vi "Create Plugin Groups.vi"(8 "error in (no error)":errorcluster, 10 "parent tag":string, 11 "Application Data In":T1) -> (0 "error out":errorcluster, 1 "async plugins tag":string, 2 "inline plugins tag":string, 3 "Application Data out":T1)   [LabVIEW 2017, in "DSF Core.lvlib"]
uses:
  DSF Core.lvlib
  Main VI/Application Data.ctl
  <vilib>/NI/Memory Manager/Classes/Pointer/Pointer.lvclass
  Classes/Framework/Framework.lvclass
  Buffer Reader/Buffer Data.ctl
  Classes/Buffer/Buffer.lvclass
  Classes/Transfer Group Status/Status.lvclass
  Typedefs/DSF Engine Framework Configuration.ctl
  Typedefs/DSF Engine Plugin Configuration.ctl
  Typedefs/DSF Timing Info.ctl
  Typedefs/DSF Engine Plugin Thread Configuration.ctl
  Typedefs/DSF Settings Info.ctl
  Typedefs/DSF Engine Transfer Group Configuration.ctl
  Typedefs/DSF Direction.ctl
  Typedefs/DSF Engine Transfer Configuration.ctl
  Typedefs/DSF Byte Order.ctl
  Typedefs/DSF Engine Channel Configuration.ctl
  Typedefs/DSF Data Type.ctl
  Typedefs/DSF Timeout Behavior.ctl
  ID to Tree Items/Tree Item Type.ctl
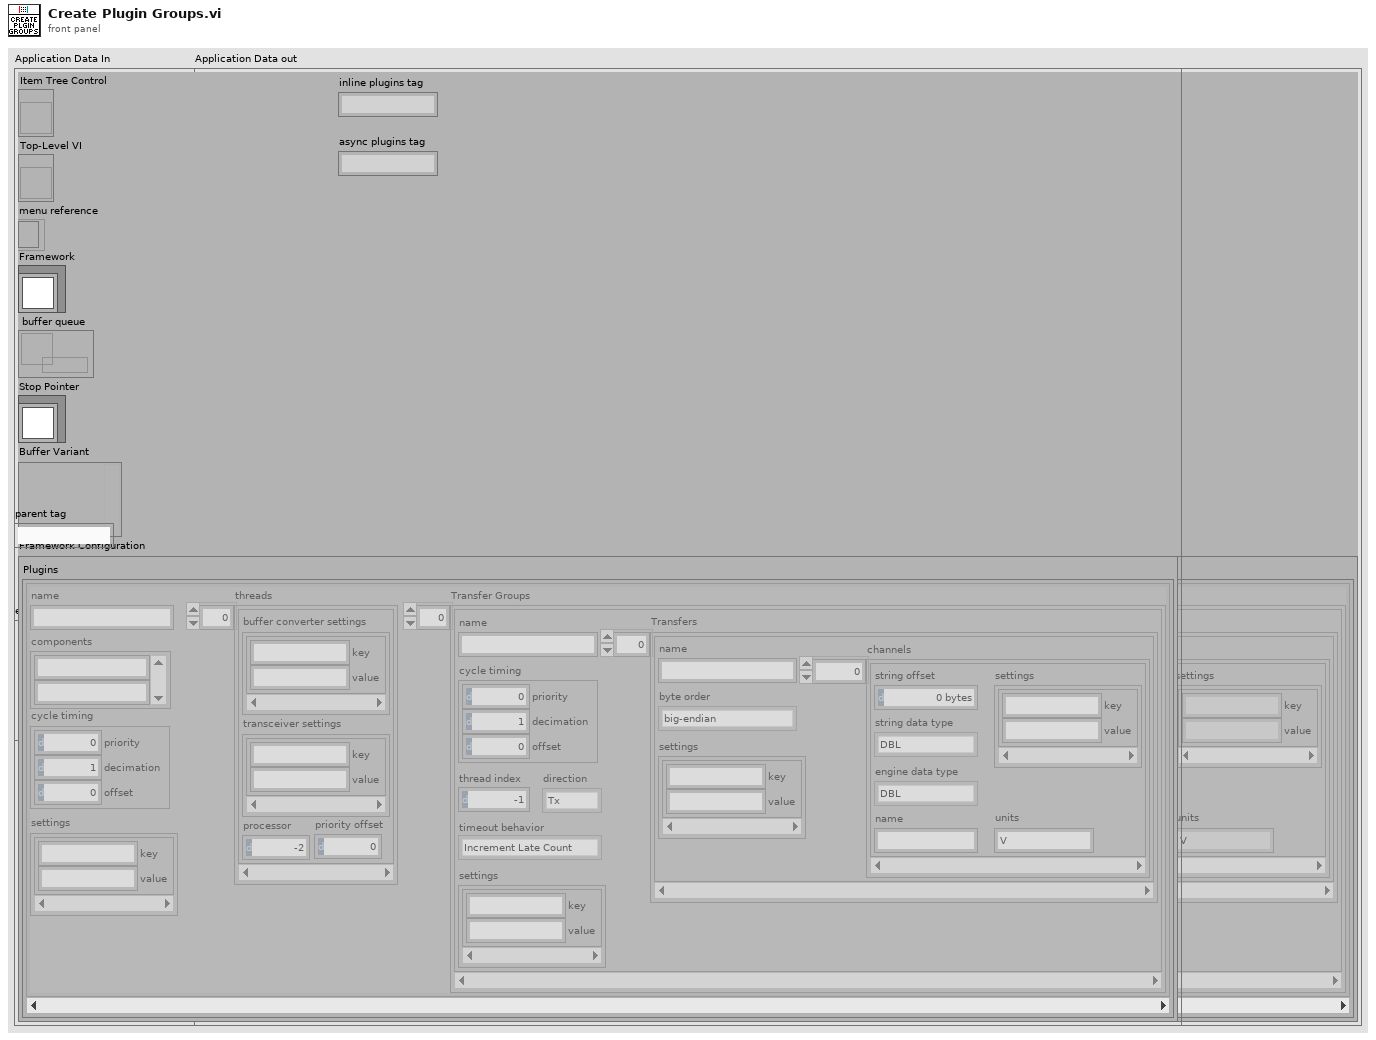
[diagram p1: front panel]
types:
  T1 = typedef "DSF Core.lvlib/Application Data.ctl" = cluster{"Item Tree Control":refnum<vi>, "Top-Level VI":refnum<vi>, "menu reference":refnum<k9>, "Framework":refnum<class "Framework.lvclass">, "buffer queue":refnum<queue>, "Stop Pointer":refnum<class "Pointer.lvclass">, "Buffer Variant":variant, "Framework Configuration":T2}
  T2 = typedef "DSF Core.lvlib/DSF Engine Framework Configuration.ctl" = cluster{"Plugins":T3[]}
  T3 = typedef "DSF Core.lvlib/DSF Engine Plugin Configuration.ctl" = cluster{"name":string, "components":string[], "cycle timing":T4, "threads":T5[], "Transfer Groups":T7[], "settings":T6}
  T4 = typedef "DSF Core.lvlib/DSF Timing Info.ctl" = cluster{"priority":u64, "decimation":u64, "offset":u64}
  T5 = typedef "DSF Core.lvlib/DSF Engine Plugin Thread Configuration.ctl" = cluster{"buffer converter settings":T6, "transceiver settings":T6, "processor":i32, "priority offset":i16}
  T6 = typedef "DSF Core.lvlib/DSF Settings Info.ctl" = cluster{"key":string, "value":string}[]
  T7 = typedef "DSF Core.lvlib/DSF Engine Transfer Group Configuration.ctl" = cluster{"name":string, "direction":T8, "cycle timing":T4, "thread index":i32, "settings":T6, "Transfers":T9[], "timeout behavior":T13}
  T8 = typedef "DSF Core.lvlib/DSF Direction.ctl" = enum8{"Tx", "Rx"}
  T9 = typedef "DSF Core.lvlib/DSF Engine Transfer Configuration.ctl" = cluster{"name":string, "byte order":T10, "settings":T6, "channels":T11[]}
  T10 = typedef "DSF Core.lvlib/DSF Byte Order.ctl" = enum8{"big-endian", "little-endian"}
  T11 = typedef "DSF Core.lvlib/DSF Engine Channel Configuration.ctl" = cluster{"string offset":u64, "string data type":T12, "engine data type":T12, "name":string, "settings":T6, "units":string}
  T12 = typedef "DSF Core.lvlib/DSF Data Type.ctl" = enum8{"Bool", "SGL", "DBL", "I8", "I16", "I32", "I64", "U8", "U16", "U32", "U64"}
  T13 = typedef "DSF Core.lvlib/DSF Timeout Behavior.ctl" = enum8{"Increment Late Count", "Throw Error"}
  T14 = typedef "DSF Core.lvlib/Buffer Data.ctl" = cluster{"Buffer":refnum<class "Buffer.lvclass">, "Status":refnum<class "Status.lvclass">, "decimation":u64, "avg bandwidth":dbl}
  T15 = typedef "DSF Core.lvlib/Tree Item Type.ctl" = enum16{"Framework", "Plugin Group", "Plugin", "Group", "Transfer", "Buffer", "Channel"}
  T16 = typedef "DSF Core.lvlib/Tree Item.ctl" = cluster{"Left Cell String":string, "Child Text":string[], "Child Tag":string, "Glyph Index":i32}
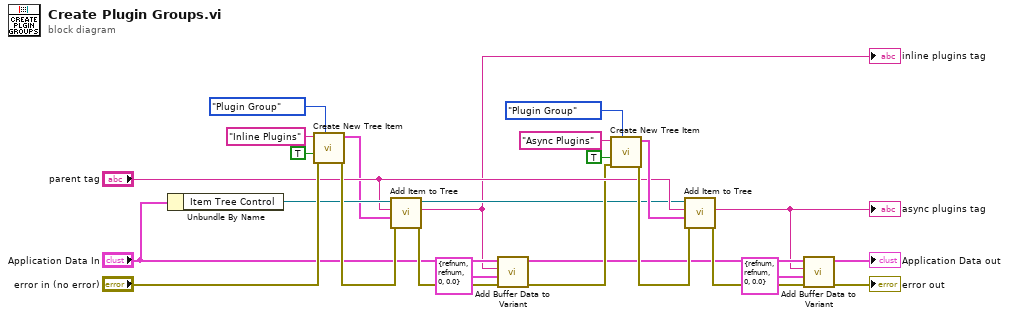
[diagram p0: block diagram]
diagram:
  n1 = Unbundle By Name("Application Data In") -> ("Item Tree Control"=w15:refnum<vi>)
  n2 = call "Create New Tree Item.vi"("Item Type"=Tree_Item_Type."Plugin Group", "error in"="error in (no error)", "found?"=TRUE, "Left Cell String"="Inline Plugins") -> ("error out"=w22:errorcluster, "Item"=w13:T16)  [unwired: 6 in]
  n3 = call "Add Item to Tree.vi"("error in (no error)"=w22, "Item"=w13, "parent tag"="parent tag", "TreeControl in"=w15) -> ("error out"=w11:errorcluster, "new item tag"=w7:string, "TreeControl out"=w8:refnum<vi>)  [unwired: 5 in]
  "inline plugins tag" <- w7
  n4 = call "Add Buffer Data to Variant.vi"("error in (no error)"=w11, "Buffer data"=T14 {"Buffer"=refnum, "Status"=refnum, "decimation"=0, "avg bandwidth"=0.0}, "tag"=w7, "Application Data In in"="Application Data In") -> ("error out"=w12:errorcluster, "Application Data In out"=w2:T1)  [unwired: 6 in]
  n5 = call "Create New Tree Item.vi"("Item Type"=Tree_Item_Type."Plugin Group", "error in"=w12, "found?"=TRUE, "Left Cell String"="Async Plugins") -> ("error out"=w18:errorcluster, "Item"=w17:T16)  [unwired: 6 in]
  n6 = call "Add Item to Tree.vi"("error in (no error)"=w18, "Item"=w17, "parent tag"="parent tag", "TreeControl in"=w8) -> ("error out"=w3:errorcluster, "new item tag"=w1:string)  [unwired: 5 in, 1 out]
  "async plugins tag" <- w1
  n7 = call "Add Buffer Data to Variant.vi"("error in (no error)"=w3, "Buffer data"=T14 {"Buffer"=refnum, "Status"=refnum, "decimation"=0, "avg bandwidth"=0.0}, "tag"=w1, "Application Data In in"=w2) -> ("error out"=→"error out":errorcluster, "Application Data In out"=→"Application Data out":T1)  [unwired: 6 in]
